vi "Normal Mode Encoder.vi"(8 "error in (no error)":errorcluster) -> (0 "error out":errorcluster)   [LabVIEW 2023, in "Encoder.lvlib"]
uses:
  Encoder.lvlib
  Internal Communication/Internal Communication.lvlib
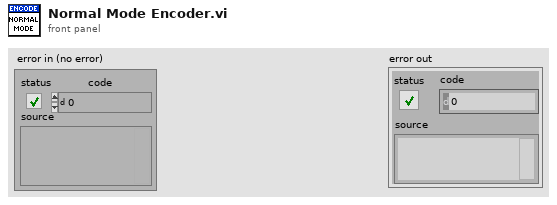
[diagram p1: front panel]
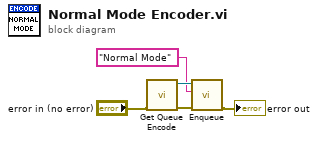
[diagram p0: block diagram]
diagram:
  n1 = call "Get Queue Encode.vi"("error in (no error)"="error in (no error)") -> ("error out"=w5:errorcluster, "Decoder Queue"=w4:refnum<queue>)  [unwired: 9 in]
  n2 = call "Enqueue.vi"("error in (no error)"=w5, "Command"="Normal Mode", "Queue In"=w4) -> ("error out"=→"error out":errorcluster)  [unwired: 7 in, 1 out]
